vi "Sorting belt control.vi"(6 "error in (no error)":errorcluster, 8 "State.Filtering":bool, 9 "Color":dbl, 10 "Baud":u32=115200, 11 "VISA Refnum in":refnum<visa-resource-name>) -> (3 "STM Feedback":string, 4 "error out":errorcluster)   [LabVIEW 2020]
doc: "This VI uses color to output sorting belt control singal.\nRemember, that your I/O device, that runs sorting belt needs to send feedback message."
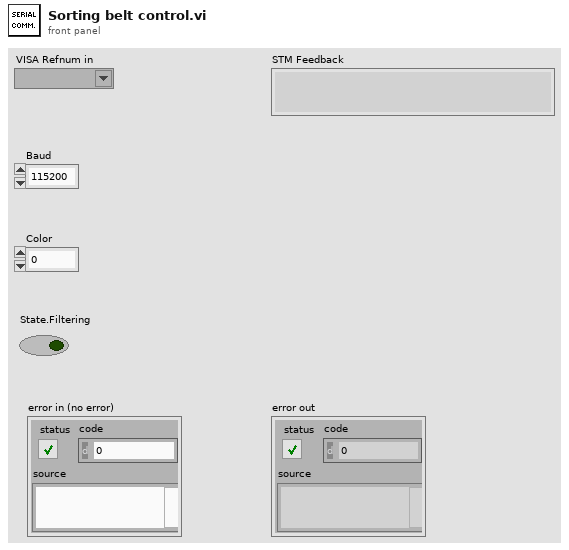
[diagram p1: front panel]
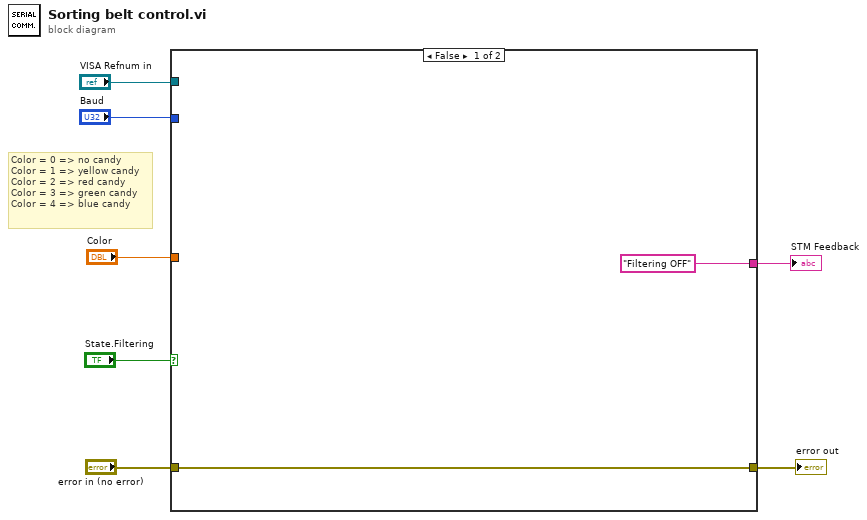
[diagram p0: block diagram]
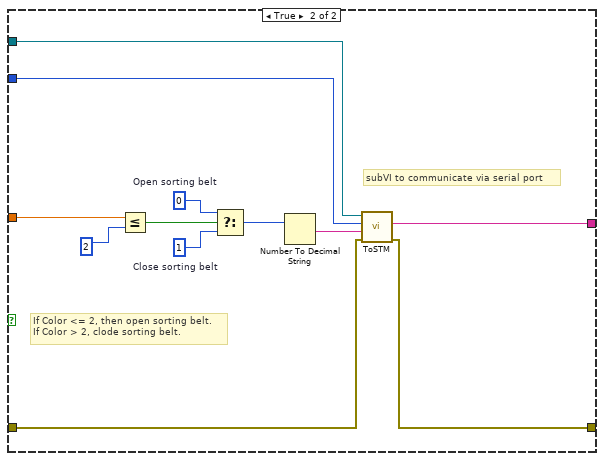
[diagram p2: hidden frame]
diagram:
  # "Color = 0 => no candy\nColor = 1 => yellow candy\nColor = 2 => red candy\nColor = 3 => green candy\nColor = 4 => blue candy"
  n1 = case shown="False" "State.Filtering" {
    tunnel: [w8 w21] -> w7
    tunnel: "error in (no error)" -> [w8 w20]
    tunnel: ["Filtering OFF" ("Feedback message") w19] -> w5
    tunnel: "Baud" -> [_ w17]
    tunnel: "VISA Refnum in" -> [_ w16]
    tunnel: "Color" -> [_ w10]
    frame False {
    }
    frame True {
      w14 = 1  # Close sorting belt
      w13 = 0  # Open sorting belt
      # "subVI to communicate via serial port"
      # "If Color <= 2, then open sorting belt.\nIf Color > 2, clode sorting belt."
      n2 = Less Or Equal?(x=w10, y=2) -> (x <= y?=w12:bool)
      n3 = Select(t=w13, s=w12, f=w14) -> (s? t:f=w15:i32)
      n4 = Number To Decimal String(number=w15) -> (decimal integer string=w18:string)  [unwired: 1 in]
      n5 = call "ToSTM.vi"("error in (no error)"=w20, "Servo position"=w18, "Baud rate"=w17, "Serial port"=w16) -> ("error out"=w21:errorcluster, "Feedback message"=w19:string)  [unwired: 5 in]
    }
  }
  "STM Feedback" <- w5
  "error out" <- w7
